vi "PH_AWG-510.ProcEvents.vi"(0 "i ref in":refnum<vi>, 5 "error in":errorcluster) -> (14 "i ref out":refnum<vi>, 19 "error out":errorcluster)   [LabVIEW 2014, in "PH_AWG-510.lvlib"]
doc: "This method is used to define the events the object will listen to. Add your own events here."
uses:
  CSCore/BaseProcess/BaseProcess.event definition.ctl
  CSCore/CAEObj/CAEObj.event definition.ctl
  CSCore/BaseProcess/BaseProcess.descriptor string definition.ctl
  PH_AWG-510.lvlib
  CSCore/BaseProcess/BaseProcess.lvlib
  CSCore/CAEObj/CAEObj.lvlib
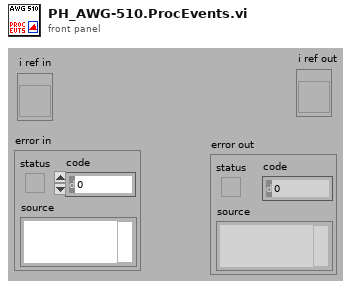
[diagram p1: front panel]
types:
  T1 = typedef "BaseProcess.lvlib/BaseProcess.event definition.ctl" = cluster{"CAEEvtDef":T2, "Data Descriptor":T3}
  T2 = typedef "CAEObj.lvlib/CAEObj.event definition.ctl" = cluster{"URL":string, "enable":bool, "ignoreResID":bool}
  T3 = typedef "BaseProcess.lvlib/BaseProcess.descriptor string definition.ctl" = string
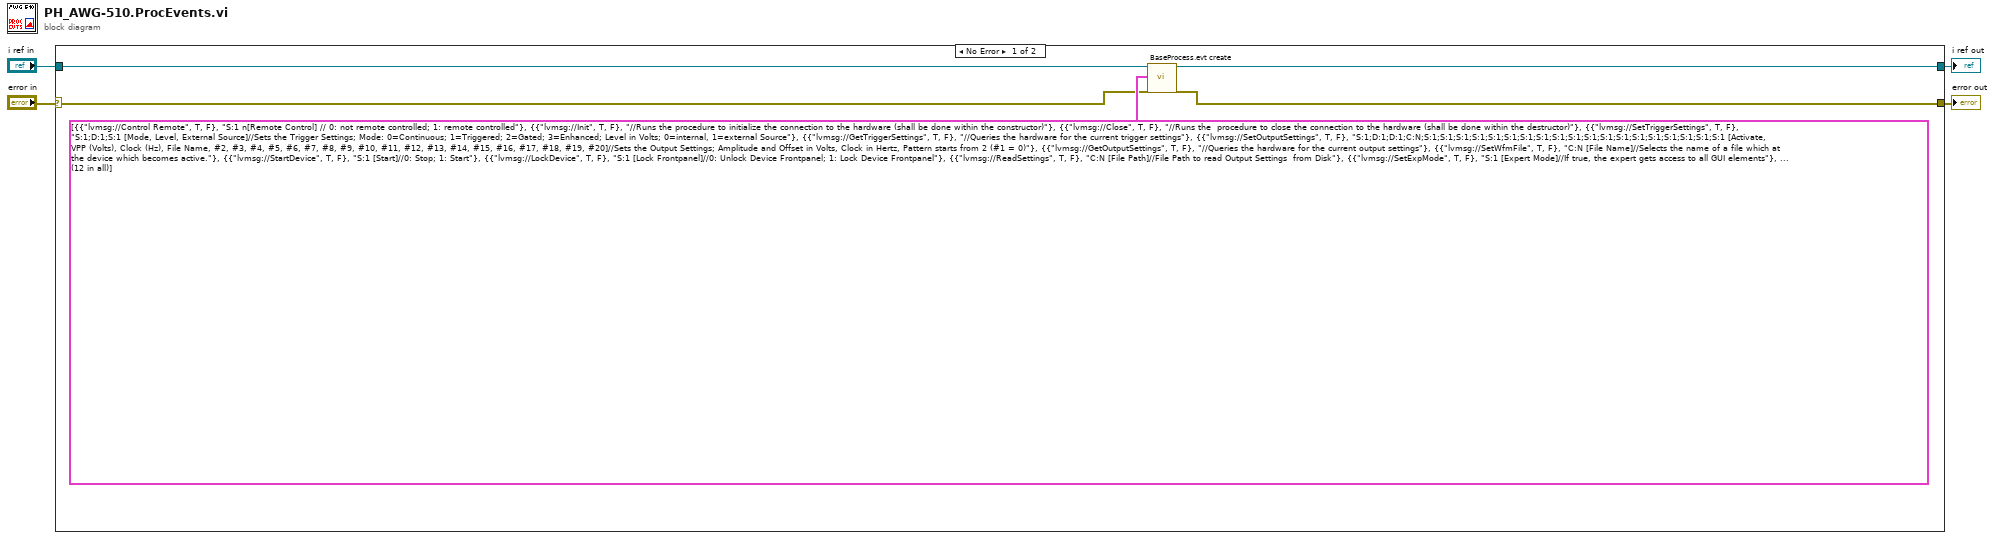
[diagram p0: block diagram]
diagram:
  n1 = case shown="No Error" "error in" {
    selector: "error in" -> [w5 w11]
    tunnel: "i ref in" -> [w9 w10]
    tunnel: [w8 w11] -> w3
    tunnel: [w7 w10] -> w2
    frame No Error {
      n2 = call "BaseProcess.evt create.vi"("i ref in"=w9, "newEvents"=T1[] [{"CAEEvtDef"={"URL"="lvmsg://Control Remote", "enable"=TRUE, "ignoreResID"=FALSE}, "Data Descriptor"="S:1 n[Remote Control] // 0: not remote controlled; 1: remote controlled"}, {"CAEEvtDef"={"URL"="lvmsg://Init", "enable"=TRUE, "ignoreResID"=FALSE}, "Data Descriptor"="//Runs the procedure to initialize the connection to the hardware (shall be done within the constructor)"}, {"CAEEvtDef"={"URL"="lvmsg://Close", "enable"=TRUE, "ignoreResID"=FALSE}, "Data Descriptor"="//Runs the  procedure to close the connection to the hardware (shall be done within the destructor)"}, {"CAEEvtDef"={"URL"="lvmsg://SetTriggerSettings", "enable"=TRUE, "ignoreResID"=FALSE}, "Data Descriptor"="S:1;D:1;S:1 [Mode, Level, External Source]//Sets the Trigger Settings; Mode: 0=Continuous; 1=Triggered; 2=Gated; 3=Enhanced; Level in Volts; 0=internal, 1=external Source"}, {"CAEEvtDef"={"URL"="lvmsg://GetTriggerSettings", "enable"=TRUE, "ignoreResID"=FALSE}, "Data Descriptor"="//Queries the hardware for the current trigger settings"}, {"CAEEvtDef"={"URL"="lvmsg://SetOutputSettings", "enable"=TRUE, "ignoreResID"=FALSE}, "Data Descriptor"="S:1;D:1;D:1;C:N;S:1;S:1;S:1;S:1;S:1;S:1;S:1;S:1;S:1;S:1;S:1;S:1;S:1;S:1;S:1;S:1;S:1;S:1;S:1 [Activate, VPP (Volts), Clock (Hz), File Name, #2, #3, #4, #5, #6, #7, #8, #9, #10, #11, #12, #13, #14, #15, #16, #17, #18, #19, #20]//Sets the Output Settings; Amplitude and Offset in Volts, Clock in Hertz, Pattern starts from 2 (#1 = 0)"}, {"CAEEvtDef"={"URL"="lvmsg://GetOutputSettings", "enable"=TRUE, "ignoreResID"=FALSE}, "Data Descriptor"="//Queries the hardware for the current output settings"}, {"CAEEvtDef"={"URL"="lvmsg://SetWfmFile", "enable"=TRUE, "ignoreResID"=FALSE}, "Data Descriptor"="C:N [File Name]//Selects the name of a file which at the device which becomes active."}, {"CAEEvtDef"={"URL"="lvmsg://StartDevice", "enable"=TRUE, "ignoreResID"=FALSE}, "Data Descriptor"="S:1 [Start]//0: Stop; 1: Start"}, {"CAEEvtDef"={"URL"="lvmsg://LockDevice", "enable"=TRUE, "ignoreResID"=FALSE}, "Data Descriptor"="S:1 [Lock Frontpanel]//0: Unlock Device Frontpanel; 1: Lock Device Frontpanel"}, {"CAEEvtDef"={"URL"="lvmsg://ReadSettings", "enable"=TRUE, "ignoreResID"=FALSE}, "Data Descriptor"="C:N [File Path]//File Path to read Output Settings  from Disk"}, {"CAEEvtDef"={"URL"="lvmsg://SetExpMode", "enable"=TRUE, "ignoreResID"=FALSE}, "Data Descriptor"="S:1 [Expert Mode]//If true, the expert gets access to all GUI elements"}] ("new events"), "error in (no error)"=w5) -> ("i ref out"=w7:refnum<vi>, "error out"=w8:errorcluster)  [unwired: 13 in, 2 out]
    }
    frame Error {
    }
  }
  "i ref out" <- w2
  "error out" <- w3
